vi "00 - Run.vi"(5 "Status Ref":refnum<vi>, 7 "Progress Bar Ref":refnum<vi>, 8 "error in (no error)":errorcluster, 10 "Global Config":T1, 11 "LabVIEW Install Folder":path) -> (0 "error out":errorcluster)   [LabVIEW 2021]
uses:
  Global Config.ctl
  ini Entry.ctl
  VIPM.ctl
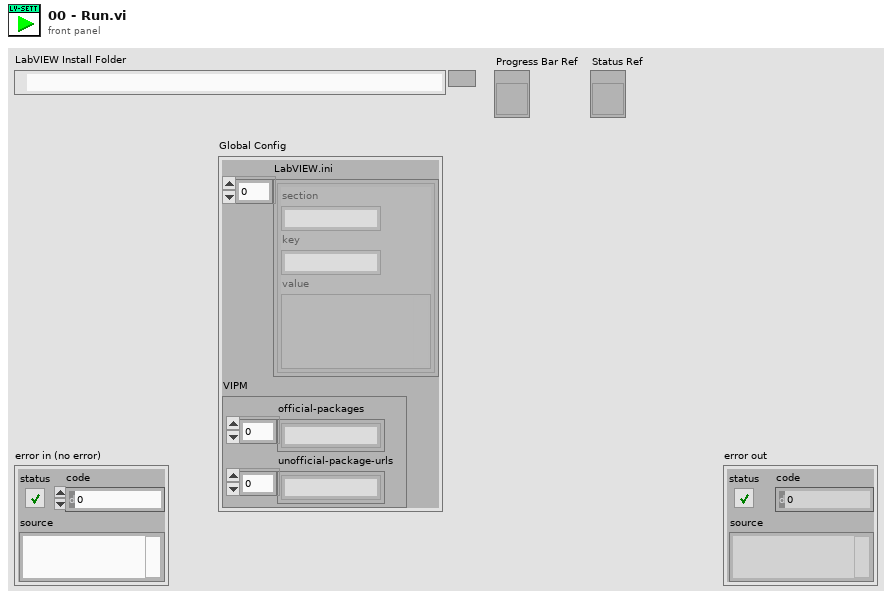
[diagram p1: front panel]
types:
  T1 = typedef "Global Config.ctl" = cluster{"LabVIEW.ini":T2[], "VIPM":T3}
  T2 = typedef "ini Entry.ctl" = cluster{"section":string, "key":string, "value":variant}
  T3 = typedef "VIPM.ctl" = cluster{"official-packages":string[], "unofficial-package-urls":string[]}
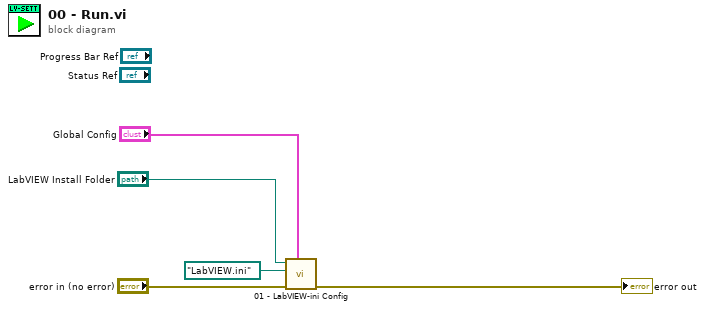
[diagram p0: block diagram]
diagram:
  n1 = call "01 - LabVIEW-ini Config.vi"("Global Config"="Global Config", "error in"="error in (no error)", "ini Name (LabVIEW.ini)"=path "LabVIEW.ini", "LabVIEW Install Folder"="LabVIEW Install Folder") -> ("error out"=→"error out":errorcluster)  [unwired: 7 in]
